vi "if_v0_v5.vi"() -> ()   [LabVIEW 2009]
panel:
  out "Solutia":dbl=3.3333333333333335
  in  "b":dbl=10.0
  in  "a":dbl=-3.0
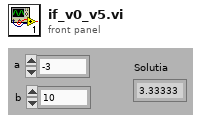
[diagram p1: front panel]
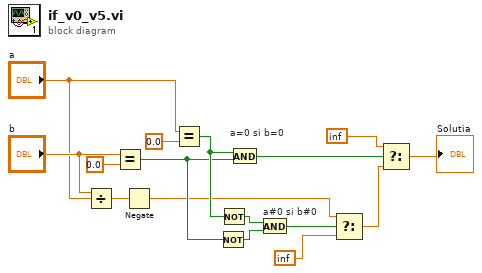
[diagram p0: block diagram]
diagram:
  n1 = Divide(x="b", y="a") -> (x/y=w4:dbl)
  n2 = Equal?(x="b", y=0.0) -> (x = y?=w9:bool)
  n3 = Negate(x=w4) -> (-x=w3:dbl)
  n4 = Equal?(x="a", y=0.0) -> (x = y?=w11:bool)
  n5 = Not(x=w9) -> (.not. x?=w8:bool)
  n6 = Not(x=w11) -> (.not. x?=w10:bool)
  n7 = And "a=0 si b=0"(x=w11, y=w9) -> (x .and. y?=w14:bool)
  n8 = And "a#0 si b#0"(x=w10, y=w8) -> (x .and. y?=w7:bool)
  n9 = Select(t=w3, s=w7, f=inf) -> (s? t:f=w1:dbl)
  n10 = Select(t=inf, s=w14, f=w1) -> (s? t:f=→"Solutia":dbl)
